vi "StringToUTF16LE.vi"(11 "ASCII":string) -> (2 "unsigned byte array":u8[](array[numeric]), 3 "Unicode":string)   [LabVIEW 2022 SP3]
uses:
  kernel32.dll
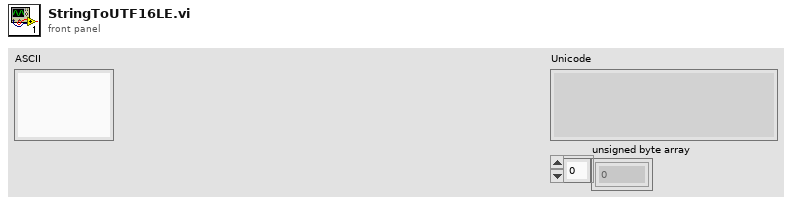
[diagram p1: front panel]
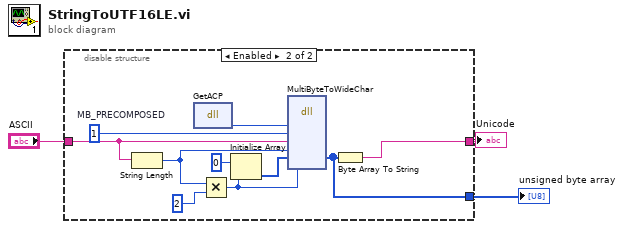
[diagram p0: block diagram]
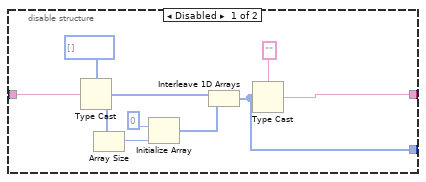
[diagram p2: hidden frame]
diagram:
  n1 = disable-structure shown="Enabled" {
    disable-tunnel: "ASCII" -> [w12 w16]
    disable-tunnel: [w5 w15] -> w2
    disable-tunnel: [w4 w13] -> w1
    frame Disabled {
      n2 = Type Cast(type=u8[] [], x=w12) -> (*(type *) &x=w8:u8[])
      n3 = Array Size(array=w8) -> (size(s)=w10:i32)
      n4 = Initialize Array(u8 0, w10) -> (w7:u8[])
      n5 = Interleave 1D Arrays(w8, w7) -> (w4:u8[])
      n6 = Type Cast(type="", x=w4) -> (*(type *) &x=w5:string)
    }
    frame Enabled {
      w21 = u32 1  # MB_PRECOMPOSED
      n7 = String Length(string=w16) -> (length=w14:i32)
      n8 = dll-call lib="kernel32.dll" fn="GetACP" label="GetACP()"() -> (w17:u32)  [unwired: 3 in, 2 out]
      n9 = Multiply(x=w14, y=2) -> (x*y=w18:i32)
      n10 = Initialize Array(u8 0, w18) -> (w19:u8[])
      n11 = dll-call lib="kernel32.dll" fn="MultiByteToWideChar"("codePage"=w17, "dwFlags"=w21, "pMultiByteStr"=w16, "cbMultiByte"=w14, "lpWideCharStr"=w19, "cchWideChar"=w18) -> ("lpWideCharStr"=w13:u8[])  [unwired: 8 in, 3 out]
      n12 = Byte Array To String(unsigned byte array=w13) -> (string=w15:string)
    }
  }
  "Unicode" <- w2
  "unsigned byte array" <- w1
